vi "ServoIDWrite.vi"(10 "ID":u8=1) -> (2 "Command":string)   [LabVIEW 2013]
panel:
  in  "IDIn":u8=1
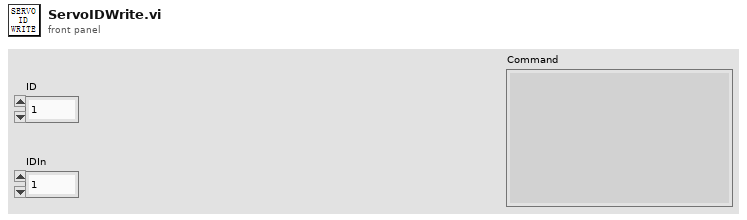
[diagram p1: front panel]
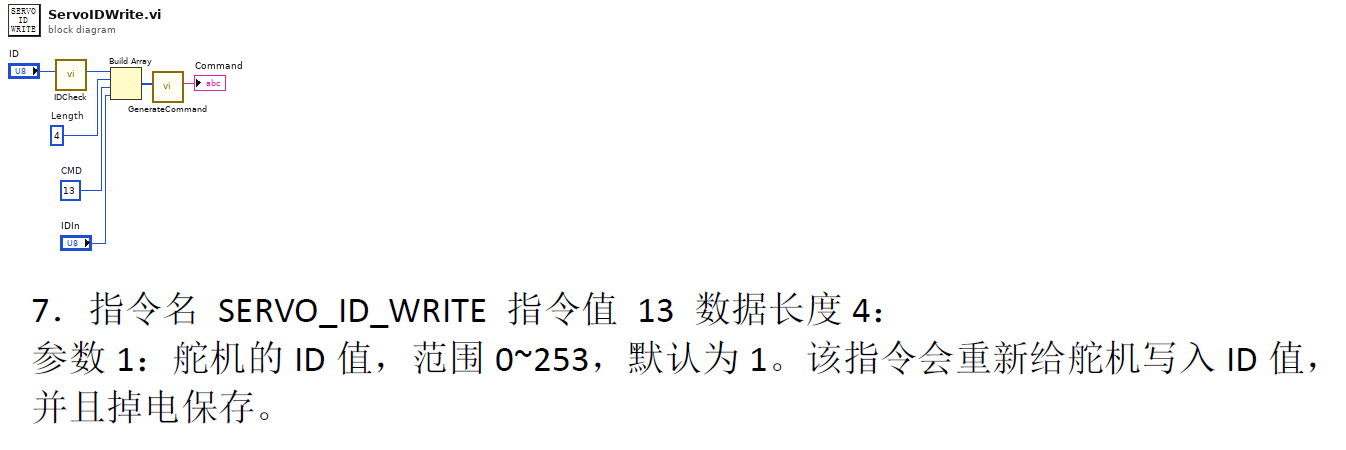
[diagram p0: block diagram]
diagram:
  w4 = u8 13  # CMD
  w5 = u8 4  # Length
  n1 = call "IDCheck.vi"("IDIn"="ID") -> ("IDOut"=w6:u8)  [unwired: 10 in]
  n2 = Build Array(w6, w5, w4, "IDIn") -> (w3:u8[])
  n3 = call "GenerateCommand.vi"("DataIn"=w3) -> ("Command"=→"Command":string)  [unwired: 10 in]
